vi "failitee.vi"() -> ()   [LabVIEW 2019]
uses:
  <vilib>/Utility/sysdir.llb/System Directory Type.ctl
panel:
  in  "system directory type":T1=1 items=["User Home"=0, "User Desktop"=1, "User Documents"=2, "User Application Data"=3, "User Preferences"=4, "User Temporary"=5, "Public Documents"=6, "Public Application Data"=7, "Public Preferences"=8, "Public Cache"=13, "System Core Libraries"=9, "System Installed Libraries"=10, "Application Files"=11, "Boot Volume Root"=12]
  out "system directory":path
  out "appended path":path
  out "name":string
  out "stripped path":path
  in  "Path":path
  out "Current VI's Path":path
  out "Default Directory":path
  out "App:Default Data Directory":path
  out "VI Library":path
  out "Application Directory":path
  out "Temporary Directory":path
  # "Build Path"
  # "Strip Path"
  # "List of Path Constants"
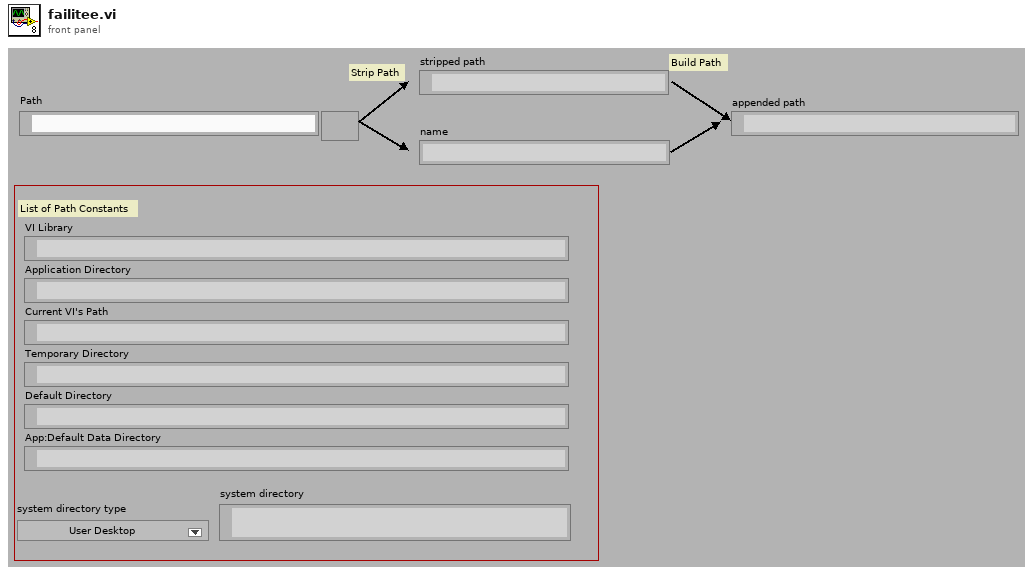
[diagram p1: front panel]
types:
  T1 = typedef "System Directory Type.ctl" = i32
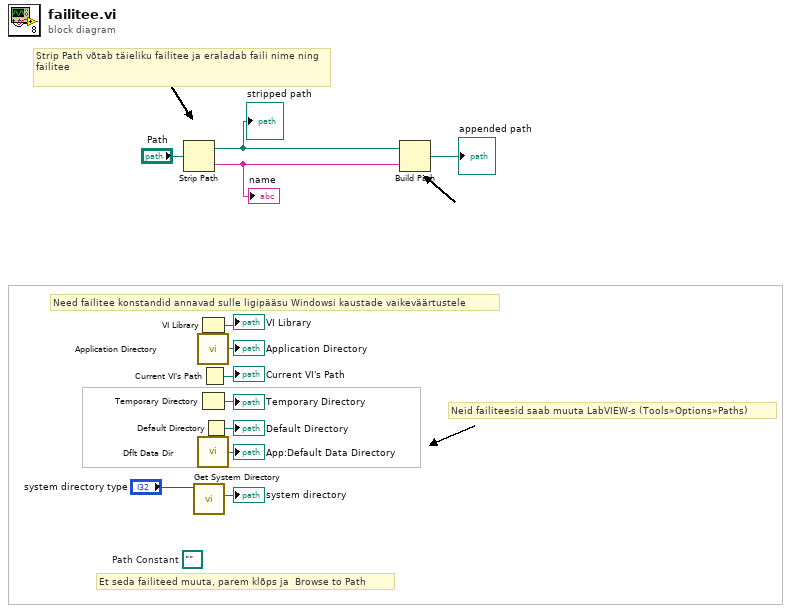
[diagram p0: block diagram]
diagram:
  (unwired) path ""  # Path Constant
  # "Neid failiteesid saab muuta LabVIEW-s (Tools»Options»Paths)"
  # "Need failitee konstandid annavad sulle ligipääsu Windowsi kaustade vaikeväärtustele"
  # "Strip Path võtab täieliku failitee ja eraladab faili nime ning failitee"
  # "Et seda failiteed muuta, parem klõps ja  Browse to Path"
  n1 = Strip Path(path="Path") -> (stripped path=w5:path, name=w4:string)
  "stripped path" <- w5
  "name" <- w4
  n2 = call <vilib>:"Get System Directory.vi"("system directory type"="system directory type") -> ("system directory"=→"system directory":path)  [unwired: 10 in]
  n3 = VI Library() -> (path=→"VI Library":path)
  n4 = call <vilib>:"Application Directory.vi"() -> ("Application Directory"=→"Application Directory":path)
  n5 = Temporary Directory() -> (→"Temporary Directory":path)
  n6 = call <vilib>:"Dflt Data Dir.vi"() -> ("App:Default Data Directory"=→"App:Default Data Directory":path)
  n7 = Current VI's Path() -> (path=→"Current VI's Path":path)
  n8 = Default Directory() -> (→"Default Directory":path)
  n9 = Build Path(base path=w5, name or relative path=w4) -> (appended path=→"appended path":path)
